vi "Read Variant Repository Tags.vi"(5 "Hide Write Once (T)":bool=TRUE, 7 "Hide Is Repository (T)":bool=TRUE, 8 "error in (no error)":errorcluster, 11 "Variant Repository In":variant) -> (0 "error out":errorcluster, 1 "Values":variant[](array[variant]), 2 "Tags":string[](array[string]), 3 "Variant Repository Out":variant, 4 "Data Types":T1[](array[typedef]))   [LabVIEW 2013]
doc: "This VI will return information about the data stored in a Variant Repository. It will return all of the <b>Tags</b> in the Variant, along with their <b>Values</b>, and <b>Data Types</b>. By default this will not show the internal tags used such as Is Variant Repository, and the Write Once tags.\n\n-------------\nBrian Hoover (Hooovahh)\n\nProduct Name: Variant Repository\nPackage File Name: lava_lib_variant_repository\nPackage Version: 1.0.1.11\nMinimum LabVIEW Version: 11.0"
uses:
  <vilib>/Utility/VariantDataType/Type.ctl
  <vilib>/Utility/VariantDataType/VariantType.lvlib
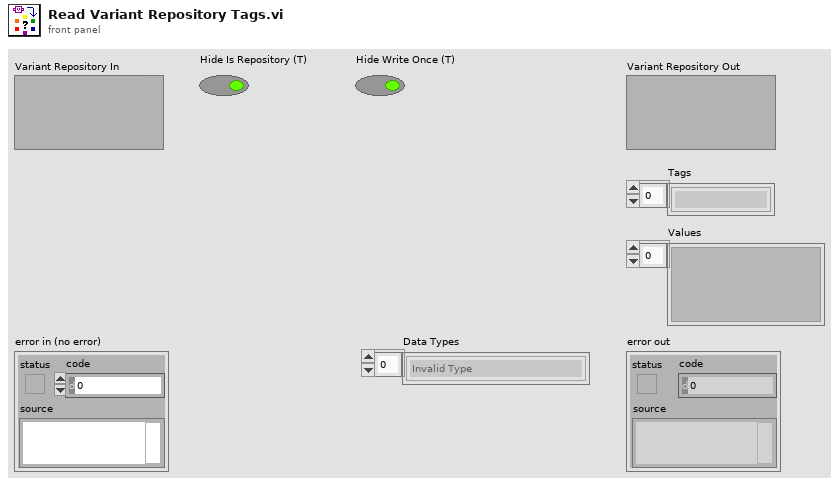
[diagram p1: front panel]
types:
  T1 = typedef "VariantType.lvlib/Type.ctl" = enum8{"Invalid Type", "Void", "I8", "I16", "I32", "I64", "U8", "U16", "U32", "U64", "Single Float", "Double Float", "Extended Float", "Single Complex", "Double Complex", "Extended Complex", "Enum U8", "Enum U16", "Enum U32", "Enum U64", "Single Float With Unit", "Double Float With Unit", "Extended Float With Unit", "Single Complex with Unit", "Double Complex with Unit", "Extended Complex with Unit", "Boolean", "String", "Path", "Picture", "Tag", "Array", "Cluster", "Variant", "LV Variant", "Waveform", "Timestamp", "Digital Waveform", "Digital Data", "ExpressData", "Refnum", "External Data", "VI", "Poly VI", "LabVIEW Class Instance", "Fixed Point"}
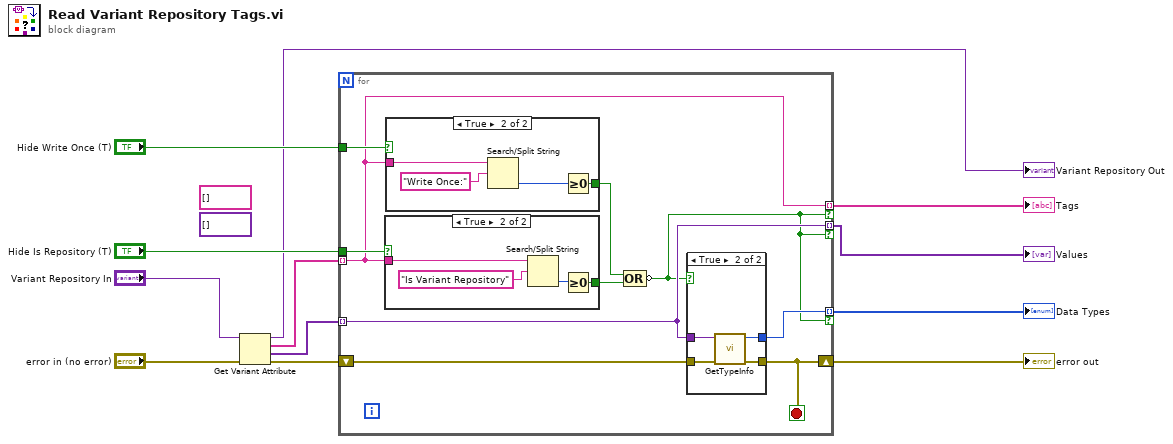
[diagram p0: block diagram]
diagram:
  (unwired) variant[] [] ("Array")
  (unwired) string[] [] ("Array")
  n1 = Get Variant Attribute(Variant="Variant Repository In", error in="error in (no error)") -> (duplicate Variant=→"Variant Repository Out":variant, names=w1:string[], values=w3:variant[], error out=w2:errorcluster)  [unwired: 2 in]
  n2 = for {
    tunnel: w3 -> [w16] mode=indexing
    shift-right: [w21] -> w12
    shift-left: w2 -> [w22]
    tunnel: w1 -> [w15] mode=indexing
    tunnel: "Hide Is Repository (T)" -> [w20]
    tunnel: "Hide Write Once (T)" -> [w19]
    tunnel: [w16] -> w6 mode=indexing if=w13
    tunnel: [w15] -> w7 mode=indexing if=w13
    tunnel: [w14] -> w4 mode=indexing if=w13
    stop <- w21 stop-if-true
    n3 = case shown="True" w20 {
      tunnel: w15 -> [_ w35]
      tunnel: [_ w32] -> w18
      frame False {
      }
      frame True {
        n4 = Search/Split String(string=w35, search string/char (-)="Is Variant Repository") -> (offset of match=w33:i32)  [unwired: 1 in, 2 out]
        n5 = Greater Or Equal To 0?(x=w33) -> (x >= 0?=w32:bool)
      }
    }
    n6 = case shown="True" w19 {
      tunnel: w15 -> [_ w31]
      tunnel: [_ w28] -> w17
      frame False {
      }
      frame True {
        n7 = Search/Split String(string=w31, search string/char (-)="Write Once:") -> (offset of match=w29:i32)  [unwired: 1 in, 2 out]
        n8 = Greater Or Equal To 0?(x=w29) -> (x >= 0?=w28:bool)
      }
    }
    n9 = Compound Arithmetic op=OR(w17, w18) -> (invert w13:bool)
    n10 = case shown="True" w13 {
      tunnel: w16 -> [_ w27]
      tunnel: w22 -> [w23 w26]
      tunnel: [w23 w25] -> w21
      tunnel: [_ w24] -> w14
      frame False {
      }
      frame True {
        n11 = call <vilib>:"GetTypeInfo.vi"("error in (no error)"=w26, "Variant"=w27) -> ("error out"=w25:errorcluster, "Type Enum"=w24:T1)  [unwired: 5 in, 3 out]
      }
    }
  }
  "error out" <- w12
  "Tags" <- w7
  "Values" <- w6
  "Data Types" <- w4
